vi "PostDataPoint.vi"(0 "InfluxDB in":refnum<class "Client.lvclass">, 5 "Database name":string, 7 "DataPoint.lvclass":refnum<class "DataPoint.lvclass">, 11 "error in (no error)":errorcluster) -> (4 "InfluxDB out":refnum<class "Client.lvclass">, 15 "error out":errorcluster)   [LabVIEW 2018, in "InfluxDB Client.lvlib" / "Client.lvclass"]
doc: "Creates a database."
uses:
  Client.lvclass
  DataPoint/DataPoint.lvclass
  DataPoint/DataPoint.lvclass/DataPoint.ctl
  RetentionPolicy/RetentionPolicy.lvclass/RetentionPolicy.ctl
  RetentionPolicy/RetentionPolicy.lvclass
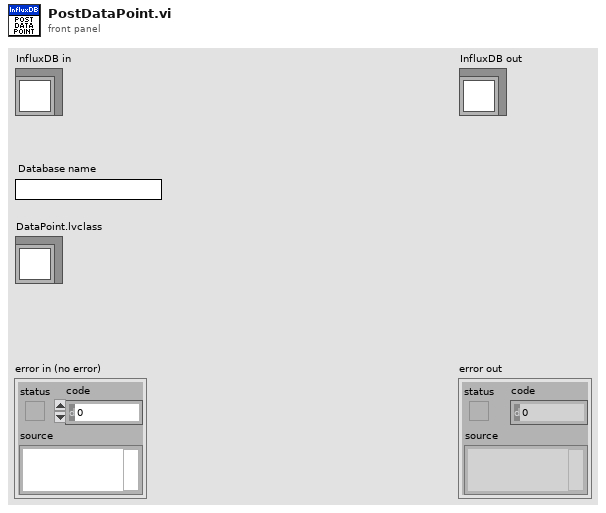
[diagram p1: front panel]
types:
  T1 = typedef "Dictionary Object RefNum__ogtk.ctl" = refnum<k1>
  T2 = typedef "InfluxDB Client.lvlib/Precision.ctl" = enum16{"Seconds", "Milliseconds", "Nanoseconds"}
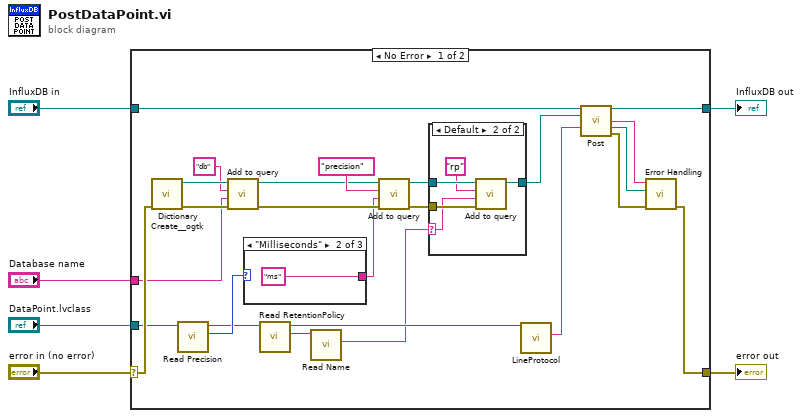
[diagram p0: block diagram]
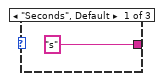
[diagram p3: hidden frame]
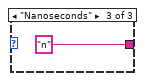
[diagram p4: hidden frame]
diagram:
  n1 = case shown="No Error" "error in (no error)" {
    selector: "error in (no error)" -> [w27 w42]
    tunnel: [w7 w42] -> w5
    tunnel: [w30 w41] -> w3
    tunnel: "InfluxDB in" -> [w31 w41]
    tunnel: "Database name" -> [w24 _]
    tunnel: "DataPoint.lvclass" -> [w20 _]
    frame No Error {
      n2 = call <userlib>:"Dictionary Create__ogtk.vi"("error in (no error)"=w27) -> ("error out"=w26:errorcluster, "dictionary out"=w29:T1)  [unwired: 9 in]
      n3 = call "Read Precision.vi"("DataPoint in"=w20) -> ("Precision"=w19:T2, "DataPoint out"=w17:refnum<class "DataPoint.lvclass">)  [unwired: 8 in, 1 out]
      n4 = call "Add to query.vi"("error in (no error)"=w26, "Value"=w24, "Parameter"="db" ("String"), "Query in"=w29) -> ("error out"=w22:errorcluster, "Query out"=w21:T1)  [unwired: 6 in]
      n5 = case shown="\"Milliseconds\"" w19 {
        tunnel: ["s" ("String") "ms" ("String") "n" ("String")] -> w18
        frame "Seconds", Default {
        }
        frame "Milliseconds" {
        }
        frame "Nanoseconds" {
        }
      }
      n6 = call "Read RetentionPolicy.vi"("DataPoint in"=w17) -> ("RetentionPolicy.lvclass"=w16:refnum<class "RetentionPolicy.lvclass">, "DataPoint out"=w15:refnum<class "DataPoint.lvclass">)  [unwired: 9 in]
      n7 = call "Read Name.vi"("RetentionPolicy in"=w16) -> ("Name"=w14:string)  [unwired: 9 in, 1 out]
      n8 = call "Add to query.vi"("error in (no error)"=w22, "Value"=w18, "Parameter"="precision" ("String"), "Query in"=w21) -> ("error out"=w12:errorcluster, "Query out"=w13:T1)  [unwired: 6 in]
      n9 = case shown="Default" w14 {
        selector: w14 -> [_ w35]
        tunnel: w13 -> [w32 w37]
        tunnel: w12 -> [_ w36]
        tunnel: [w32 w33] -> w11
        frame "" {
        }
        frame Default {
          n10 = call "Add to query.vi"("error in (no error)"=w36, "Value"=w35, "Parameter"="rp" ("String"), "Query in"=w37) -> ("Query out"=w33:T1)  [unwired: 6 in, 1 out]
        }
      }
      n11 = call "LineProtocol.vi"("DataPoint in"=w15) -> ("Line protocol"=w25:string)  [unwired: 8 in, 2 out]
      n12 = call "Post.vi"("InfluxDB Client in"=w31, "Query"=w11, "buffer"=w25) -> ("InfluxDB Client out"=w30:refnum<class "Client.lvclass">, "Status code"=w10:string, "Headers"=w9:T1, "error out"=w8:errorcluster)  [unwired: 8 in, 1 out]
      n13 = call "Error Handling.vi"("error in (no error)"=w8, "HTTP headers"=w9, "HTTP status code"=w10) -> ("error out"=w7:errorcluster)  [unwired: 8 in]
    }
    frame Error {
    }
  }
  "error out" <- w5
  "InfluxDB out" <- w3
